vi "Z_ReflectorPosition_RT.vi"(9 "ReturnDataStatus":T1, 10 "ReflectorPosition":i32) -> (2 "Command":string)   [LabVIEW 2017]
uses:
  sobot structures/ReturnDataStatus.ctl
  sobot structures/SoBot_CommandTypes.ctl
  sobot structures/Z_Command.ctl
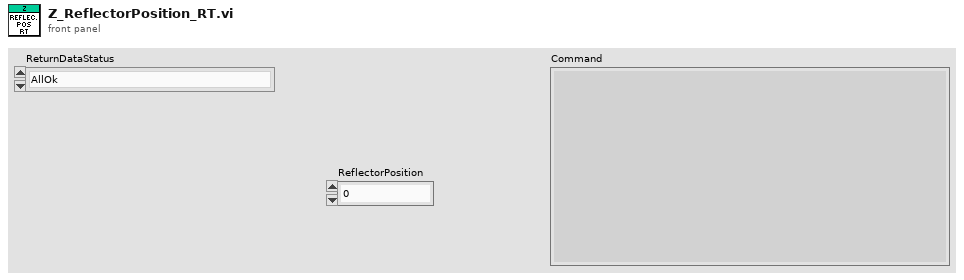
[diagram p1: front panel]
types:
  T1 = typedef "ReturnDataStatus.ctl" = enum16{"AllOk", "Error"}
  T2 = typedef "Z_Command.ctl" = enum16{"Z_Initialize", "Z_MoveToPosition", "Z_Focus", "Z_ReflectorPosition"}
  T3 = typedef "SoBot_CommandTypes.ctl" = enum16{"General_Command", "XY_Command", "Z_Command", "Plattform_Command"}
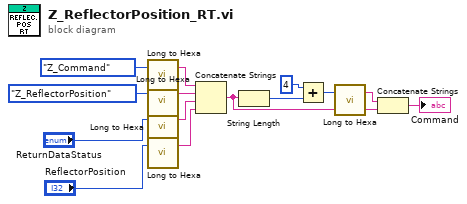
[diagram p0: block diagram]
diagram:
  n1 = call "Long to Hexa.vi"("Long"=SoBot_CommandTypes."Z_Command" ("SoBot_CommandTypes")) -> ("Hexa"=w14:string)  [unwired: 2 in]
  n2 = call "Long to Hexa.vi"("Long"=Z_Command."Z_ReflectorPosition" ("Z_Command")) -> ("Hexa"=w13:string)  [unwired: 2 in]
  n3 = call "Long to Hexa.vi"("Long"="ReturnDataStatus") -> ("Hexa"=w3:string)  [unwired: 2 in]
  n4 = call "Long to Hexa.vi"("Long"="ReflectorPosition") -> ("Hexa"=w2:string)  [unwired: 2 in]
  n5 = Concatenate Strings(w14, w13, w3, w2) -> (w8:string)
  n6 = String Length(string=w8) -> (length=w12:i32)
  n7 = Add(x=4, y=w12) -> (x+y=w10:i32)
  n8 = call "Long to Hexa.vi"("Long"=w10) -> ("Hexa"=w9:string)  [unwired: 2 in]
  n9 = Concatenate Strings(w9, w8) -> (→"Command":string)
